vi "ReadAndSaveTemperature.vi"(0 "object in":refnum<class "TC0608.lvclass">, 2 "tdms file":refnum<k34>, 5 "error in (no error)":errorcluster) -> (14 "object out":refnum<class "TC0608.lvclass">, 16 "temperature (C)":dbl, 19 "error out":errorcluster)   [LabVIEW 2023, in "TC0608.lvclass"]
uses:
  TC0608.lvclass
  TC0608.lvclass/TC0608.ctl
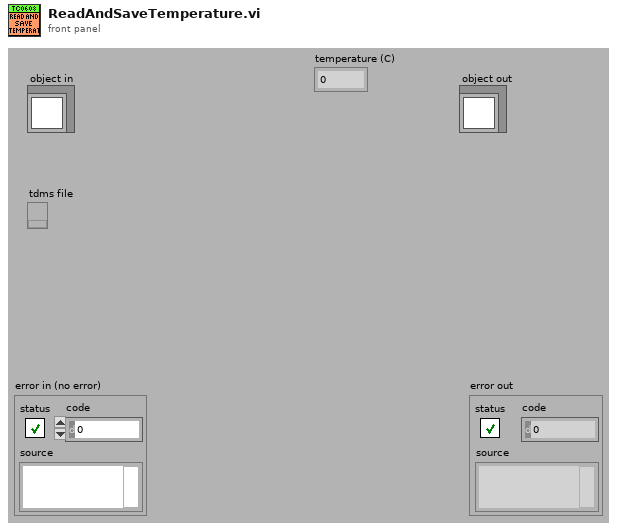
[diagram p1: front panel]
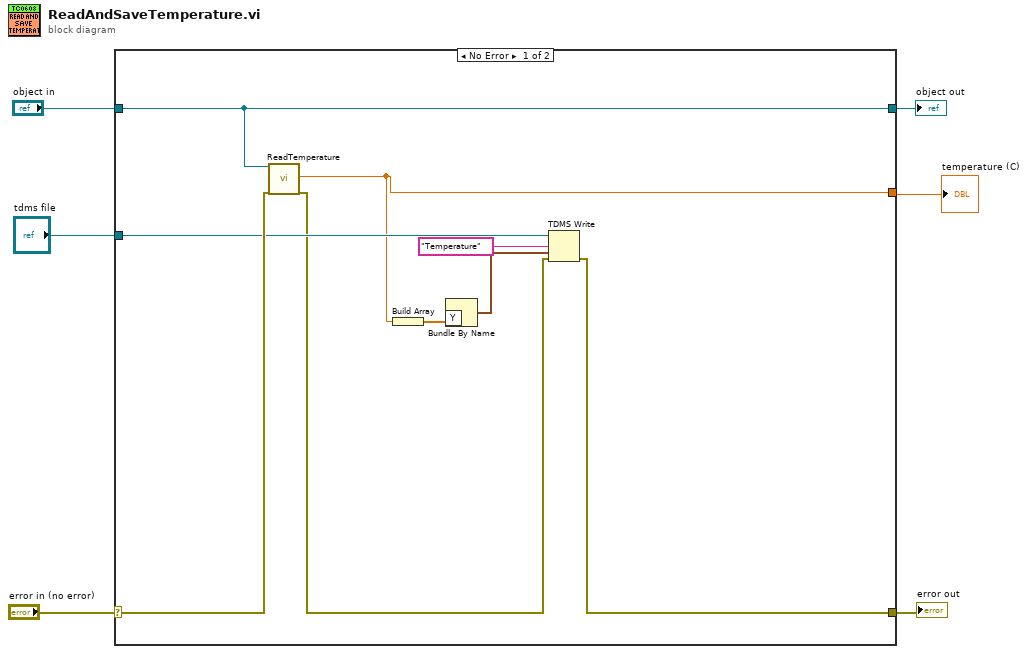
[diagram p0: block diagram]
diagram:
  n1 = case shown="No Error" "error in (no error)" {
    selector: "error in (no error)" -> [w14 w17]
    tunnel: [w8 w17] -> w5
    tunnel: [w15 w16] -> w3
    tunnel: "object in" -> [w15 w16]
    tunnel: "tdms file" -> [w13 _]
    tunnel: [w7 _] -> w1
    frame No Error {
      n2 = call-dynamic "ReadTemperature.vi"("object in"=w15, "error in (no error)"=w14) -> ("temperature (C)"=w7:dbl, "error out"=w9:errorcluster)  [unwired: 15 in, 1 out]
      n3 = Build Array(w7) -> (w12:dbl[])
      n4 = Bundle By Name("Y"=w12) -> (w11:waveform(dbl))  [unwired: 1 in]
      n5 = TDMS Write(0:w13, 7:"Temperature" ("channel name(s) in (Untitled)"), 9:w11, 11:w9) -> (15:w8:errorcluster)  [unwired: 2 in, 3 out]
    }
    frame Error {
    }
  }
  "error out" <- w5
  "object out" <- w3
  "temperature (C)" <- w1
